vi "calculator.vi"() -> ()   [LabVIEW 2022 SP3]
panel:
  in  "Calculator display":string
  in  "Calculator UI":T1
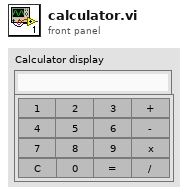
[diagram p1: front panel]
types:
  T1 = cluster{"1":bool, "2":bool, "3":bool, "4":bool, "5":bool, "6":bool, "7":bool, "8":bool, "9":bool, "0":bool, "Add":bool, "Sub":bool, "Multiply":bool, "Divide":bool, "Clear":bool, "Result":bool}
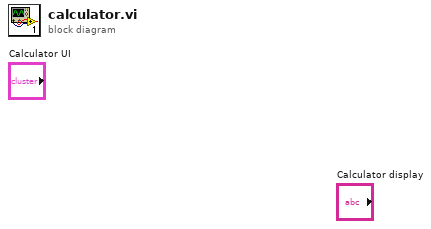
[diagram p0: block diagram]
diagram:
